vi "Generate EIS Plots.vi"(8 "error in (no error)":errorcluster, 10 "EIS Parameters":T1={"EIS Mode"=2, "EIS DC Potential"=650.0, "EIS Start Frequency"=1000.0, "EIS Stop Frequency"=500.0, "EIS Delta Frequency"=100.0, "EIS DC Current"=0.0, "AC Signal (mV/mA RMS)"=20.0, "Cycles at Frequency"=5.0, "EIS AC Step Delay"=1.0} {"EIS Mode" items=["Voltage (PEIS)"=1, "Current (GEIS)"=2]}, 11 "TDMS Data File":path) -> (0 "error out":errorcluster, 1 "EIS Bode Magnitude":cluster{dbl[], dbl[]}(graph), 2 "EIS Bode Phase":cluster{dbl[], dbl[]}(graph), 3 "EIS Nyquist":cluster{dbl[], dbl[]}(graph))   [LabVIEW 2023, in "ACIR_EIS.lvclass"]
uses:
  EIS Parameters.ctl
  EIS Mode.ctl
  <vilib>/Analysis/baseanly.llb/Mean (DBL).vi
  <vilib>/Analysis/2dsp.llb/Real FFT.vi
  ACIR_EIS.lvclass
  ACIR_EIS.lvclass/ACIR_EIS.ctl
  <vilib>/Analysis/NI_AALBase.lvlib
  <vilib>/Analysis/NI_AALPro.lvlib
panel:
  out "frequencies":dbl[](array[numeric])
  out "dF":dbl
  out "frequency (hz)":dbl
  out "period (seconds)":dbl format="%#_6f"
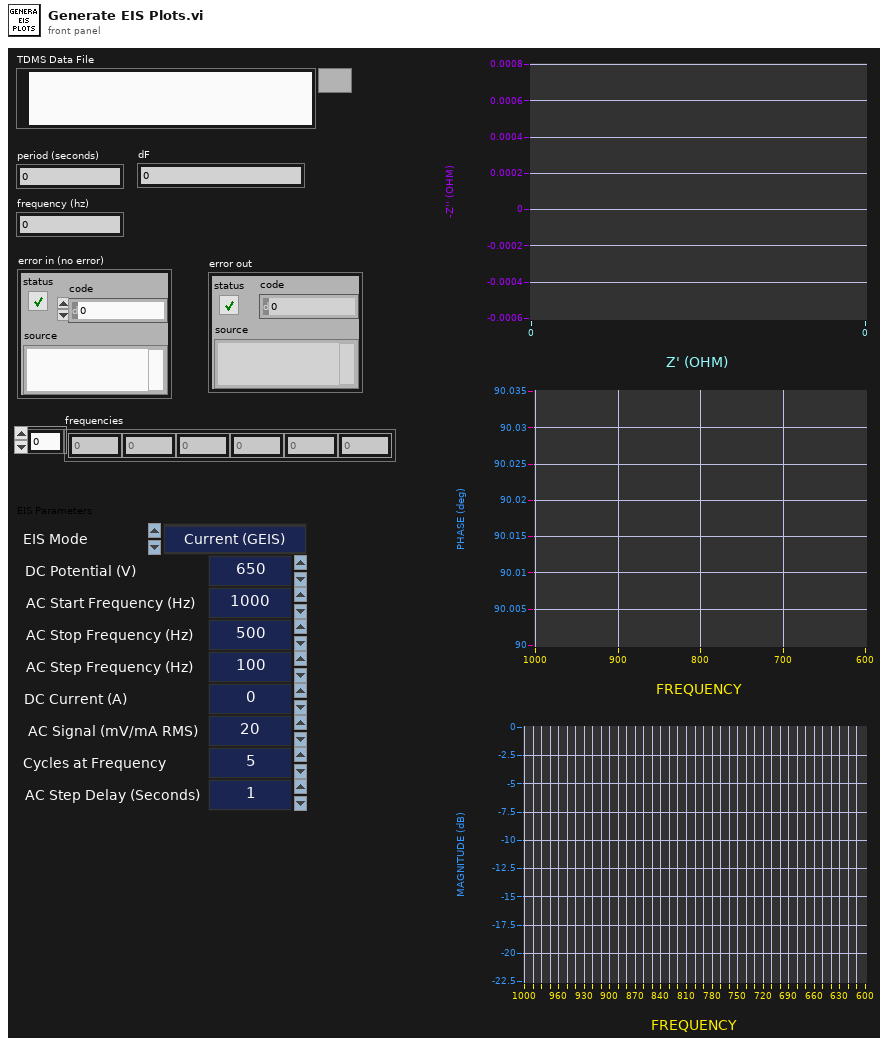
[diagram p1: front panel]
types:
  T1 = typedef "ACIR_EIS.lvclass/EIS Parameters.ctl" = cluster{"EIS Mode":T2, "EIS DC Potential":dbl, "EIS Start Frequency":dbl, "EIS Stop Frequency":dbl, "EIS Delta Frequency":dbl, "EIS DC Current":dbl, "AC Signal (mV/mA RMS)":dbl, "Cycles at Frequency":dbl, "EIS AC Step Delay":dbl}
  T2 = typedef "ACIR_EIS.lvclass/EIS Mode.ctl" = u16
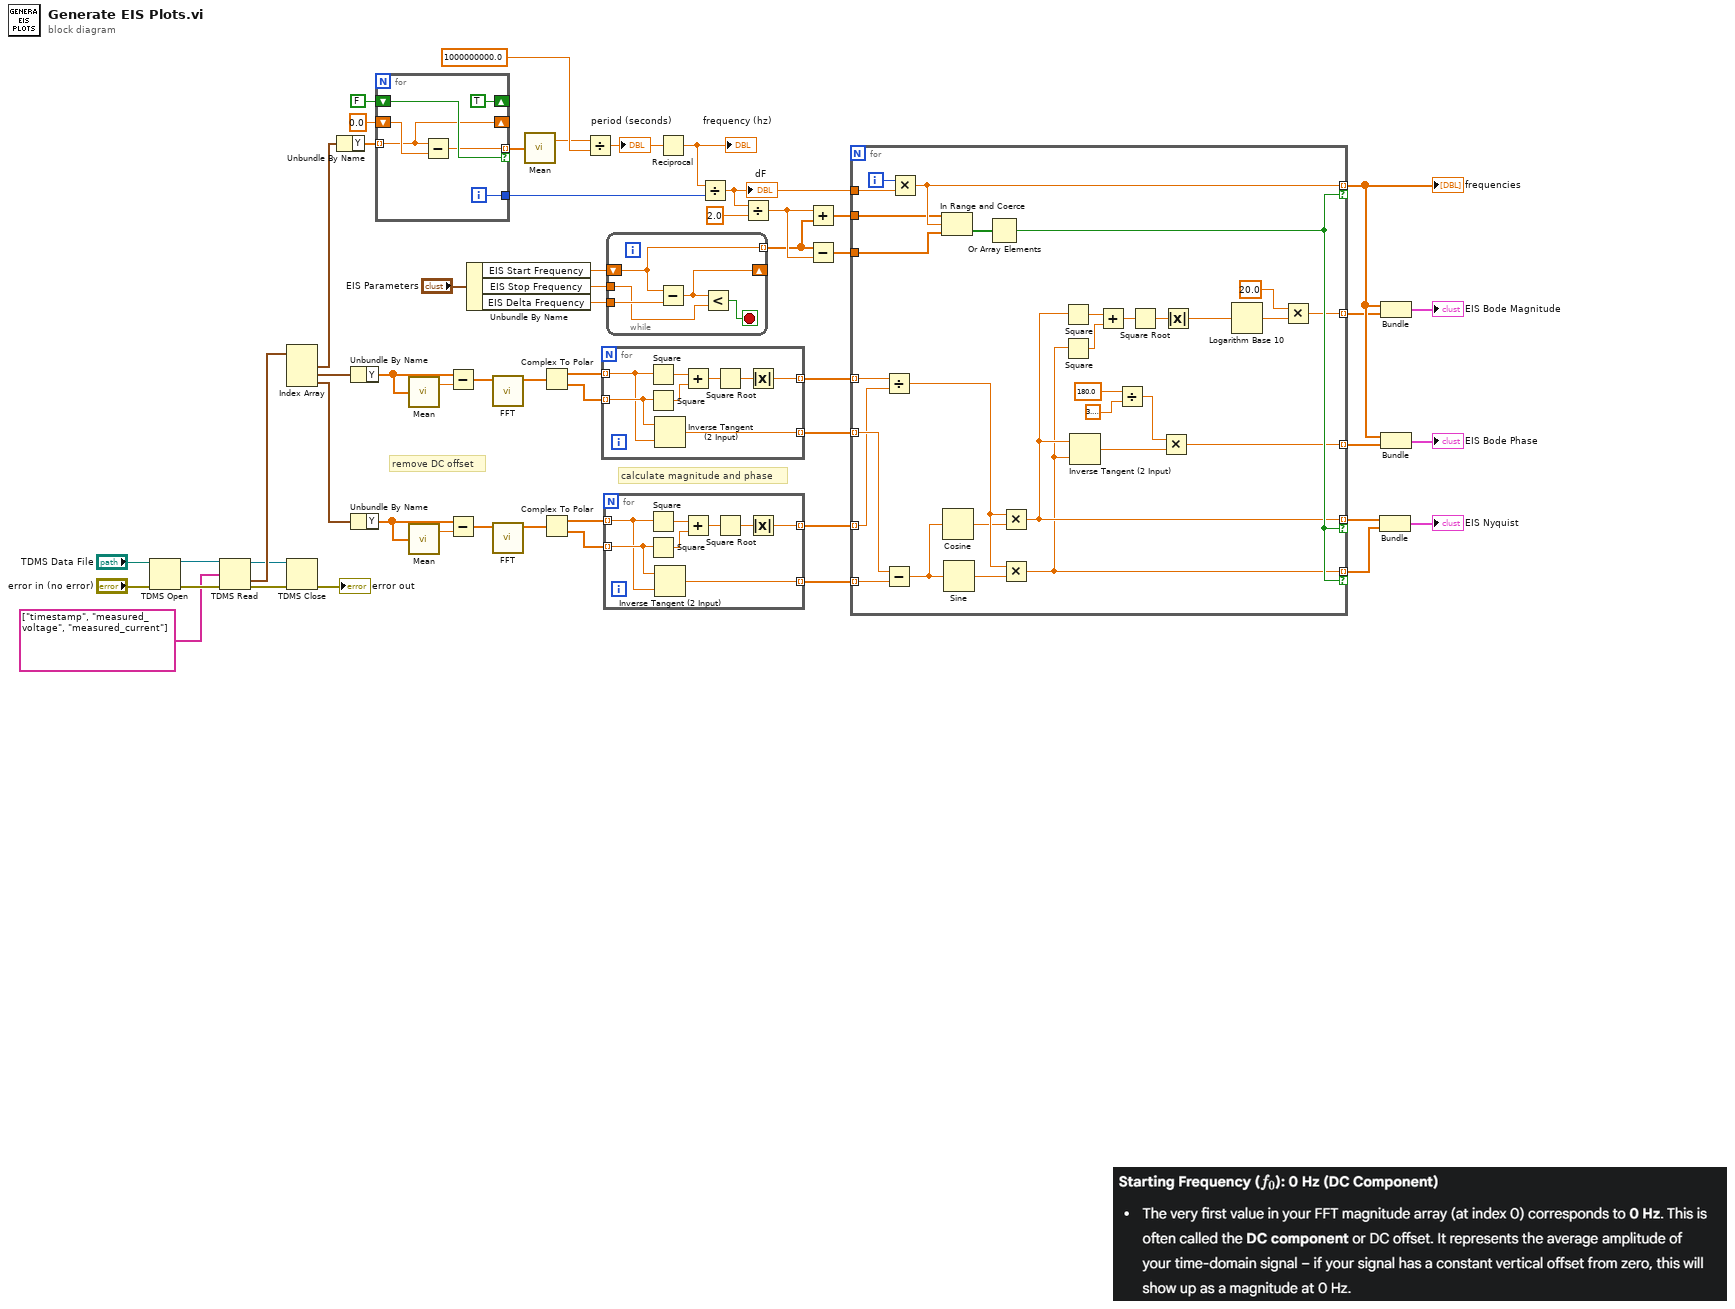
[diagram p0: block diagram]
diagram:
  # "calculate magnitude and phase"
  # "remove DC offset"
  n1 = TDMS Open(8:"error in (no error)", 11:"TDMS Data File") -> (0:w53:errorcluster, 3:w52:refnum<k34>)  [unwired: 5 in]
  n2 = TDMS Read(0:w52, 7:string[] ["timestamp", "measured_voltage", "measured_current"] ("channel name(s) in"), 11:w53) -> (4:w34:refnum<k34>, 10:w50:waveform(dbl)[], 15:w35:errorcluster)  [unwired: 5 in, 3 out]
  n3 = Index Array(array=w50) -> (element #1=w49:waveform(dbl), element #2=w40:waveform(dbl), element #3=w42:waveform(dbl))  [unwired: 3 in]
  n4 = TDMS Close(8:w35, 11:w34) -> (0:→"error out":errorcluster)  [unwired: 1 out]
  n5 = Unbundle By Name(w49) -> ("Y"=w48:dbl[])
  n6 = Unbundle By Name(w40) -> ("Y"=w30:dbl[])
  n7 = Unbundle By Name(w42) -> ("Y"=w26:dbl[])
  n8 = for {
    tunnel: w48 -> [w58] mode=indexing
    tunnel: [w57] -> w46 mode=indexing if=w60
    shift-right: [w58] -> _
    shift-left: 0.0 -> [w59]
    shift-right: [TRUE] -> _
    shift-left: FALSE -> [w60]
    tunnel: [w56] -> w22
    i -> [w56]
    n9 = Subtract(x=w58, y=w59) -> (x-y=w57:dbl)
  }
  n10 = call-poly <vilib>:"Mean.vi"("X"=w30) -> ("mean"=w29:dbl)  [unwired: 1 out]
  n11 = call-poly <vilib>:"Mean.vi"("X"=w26) -> ("mean"=w27:dbl)  [unwired: 1 out]
  n12 = Subtract(x=w30, y=w29) -> (x-y=w28:dbl[])
  n13 = Subtract(x=w26, y=w27) -> (x-y=w25:dbl[])
  n14 = Unbundle By Name("EIS Parameters") -> ("EIS Start Frequency"=w2:dbl, "EIS Stop Frequency"=w3:dbl, "EIS Delta Frequency"=w4:dbl)
  n15 = call-poly <vilib>:"FFT.vi"("X"=w28) -> ("FFT {X}"=w21:cdb[])  [unwired: 9 in, 1 out]
  n16 = call-poly <vilib>:"FFT.vi"("X"=w25) -> ("FFT {X}"=w41:cdb[])  [unwired: 9 in, 1 out]
  n17 = call-poly <vilib>:"Mean.vi"("X"=w46) -> ("mean"=w45:dbl)  [unwired: 1 out]
  n18 = Complex To Polar(r * e^(i*theta)=w21) -> (r=w20:dbl[], theta=w36:dbl[])
  n19 = Complex To Polar(r * e^(i*theta)=w41) -> (r=w19:dbl[], theta=w39:dbl[])
  n20 = Divide(x=w45, y=1000000000.0) -> (x/y=w38:dbl)
  "period (seconds)" <- w38
  n21 = for {
    tunnel: w20 -> [w63] mode=indexing
    tunnel: w36 -> [w64] mode=indexing
    tunnel: [w65] -> w24 mode=indexing
    tunnel: [w62] -> w32 mode=indexing
    n22 = Square(x=w63) -> (x^2=w69:dbl)
    n23 = Square(x=w64) -> (x^2=w68:dbl)
    n24 = Inverse Tangent (2 Input)(1:w63, 2:w64) -> (0:w62:dbl)
    n25 = Add(x=w69, y=w68) -> (x+y=w67:dbl)
    n26 = Square Root(x=w67) -> (sqrt(x)=w66:dbl)
    n27 = Absolute Value(x=w66) -> (abs(x)=w65:dbl)
  }
  n28 = for {
    tunnel: w19 -> [w71] mode=indexing
    tunnel: w39 -> [w72] mode=indexing
    tunnel: [w73] -> w37 mode=indexing
    tunnel: [w70] -> w31 mode=indexing
    n29 = Square(x=w71) -> (x^2=w77:dbl)
    n30 = Square(x=w72) -> (x^2=w76:dbl)
    n31 = Inverse Tangent (2 Input)(1:w71, 2:w72) -> (0:w70:dbl)
    n32 = Add(x=w77, y=w76) -> (x+y=w75:dbl)
    n33 = Square Root(x=w75) -> (sqrt(x)=w74:dbl)
    n34 = Absolute Value(x=w74) -> (abs(x)=w73:dbl)
  }
  n35 = while {
    tunnel: w4 -> [w82]
    tunnel: w3 -> [w81]
    shift-right: [w80] -> _
    shift-left: w2 -> [w79]
    tunnel: [w79] -> w1 mode=indexing
    stop <- w78 stop-if-true
    n36 = Subtract(x=w79, y=w82) -> (x-y=w80:dbl)
    n37 = Less?(x=w80, y=w81) -> (x < y?=w78:bool)
  }
  n38 = Reciprocal(x=w38) -> (1/x=w23:dbl)
  "frequency (hz)" <- w23
  n39 = Divide(x=w23, y=w22) -> (x/y=w18:dbl)
  "dF" <- w18
  n40 = Divide(x=w18, y=2.0) -> (x/y=w16:dbl)
  n41 = Add(x=w16, y=w1) -> (x+y=w14:dbl[])
  n42 = Subtract(x=w1, y=w16) -> (x-y=w15:dbl[])
  n43 = for {
    tunnel: w24 -> [w107] mode=indexing
    tunnel: w37 -> [w105] mode=indexing
    tunnel: w32 -> [w106] mode=indexing
    tunnel: w31 -> [w108] mode=indexing
    tunnel: [w89] -> w12 mode=indexing if=w98
    tunnel: [w88] -> w11 mode=indexing if=w98
    tunnel: w18 -> [w104]
    tunnel: [w102] -> w8 mode=indexing if=w98
    tunnel: w15 -> [w100]
    tunnel: w14 -> [w101]
    tunnel: [w90] -> w7 mode=indexing
    tunnel: [w83] -> w6 mode=indexing
    i -> [w103]
    n44 = Divide(x=w107, y=w105) -> (x/y=w110:dbl)
    n45 = Subtract(x=w106, y=w108) -> (x-y=w112:dbl)
    n46 = Multiply(x=w103, y=w104) -> (x*y=w102:dbl)
    n47 = In Range and Coerce(upper limit=w101, x=w102, lower limit=w100) -> (In Range?=w99:bool[])  [unwired: 1 out]
    n48 = Cosine(x=w112) -> (cos(x)=w109:dbl)
    n49 = Sine(x=w112) -> (sin(x)=w111:dbl)
    n50 = Or Array Elements(Boolean array=w99) -> (logical OR=w98:bool)
    n51 = Multiply(x=w110, y=w109) -> (x*y=w89:dbl)
    n52 = Multiply(x=w110, y=w111) -> (x*y=w88:dbl)
    n53 = Square(x=w89) -> (x^2=w94:dbl)
    n54 = Square(x=w88) -> (x^2=w95:dbl)
    n55 = Inverse Tangent (2 Input)(1:w88, 2:w89) -> (0:w87:dbl)
    n56 = Add(x=w94, y=w95) -> (x+y=w96:dbl)
    n57 = Divide(x=180.0 ("y"), y=3.141592653589793) -> (x/y=w84:dbl)
    n58 = Square Root(x=w96) -> (sqrt(x)=w97:dbl)
    n59 = Multiply(x=w84, y=w87) -> (x*y=w83:dbl)
    n60 = Absolute Value(x=w97) -> (abs(x)=w91:dbl)
    n61 = Logarithm Base 10(1:w91) -> (0:w92:dbl)
    n62 = Multiply(x=20.0 ("y"), y=w92) -> (x*y=w90:dbl)
  }
  "frequencies" <- w8
  n63 = Bundle(w12, w11) -> (→"EIS Nyquist":cluster{dbl[], dbl[]})  [unwired: 1 in]
  n64 = Bundle(w8, w7) -> (→"EIS Bode Magnitude":cluster{dbl[], dbl[]})  [unwired: 1 in]
  n65 = Bundle(w8, w6) -> (→"EIS Bode Phase":cluster{dbl[], dbl[]})  [unwired: 1 in]
